vi "Stop Core.vi"(10 "final error code":i32, 11 "Nested in":refnum<class "Valve.lvclass">) -> (3 "Nested out":refnum<class "Valve.lvclass">)   [LabVIEW 2021, in "Valve.lvlib" / "Valve.lvclass"]
doc: "(<B>Filename</B>: Actor Framework.lvlib:Actor.lvclass:Stop Core.vi)\n\nDefines what the actor does before it stops. Use the <B>final error code</B> input to determine whether the actor shut down in response to an error.\n\nBy default, this method does nothing. A descendant class may override it to define behavior, such as shutting down any processes the actor initiated in its override of the Actor Core method."
uses:
  Valve.lvclass
  Valve.lvclass/Valve.ctl
  <vilib>/MGI/Panel Manager/Panel Actor/Panel Actor/Panel Actor.lvclass
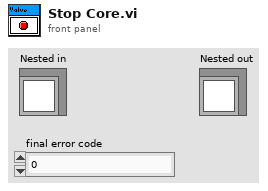
[diagram p1: front panel]
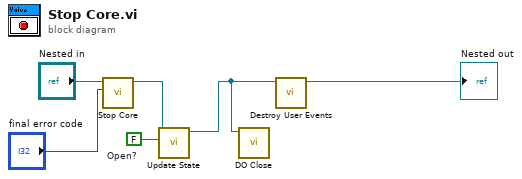
[diagram p0: block diagram]
diagram:
  w1 = FALSE  # Open?
  n1 = call-parent "Stop Core.vi"("final error code"="final error code", "Actor in"="Nested in") -> ("Actor out"=w3:refnum<class "Valve.lvclass">)  [unwired: 9 in]
  n2 = call "Update State.vi"("Open?"=w1, "Valve in"=w3) -> ("Valve out"=w2:refnum<class "Valve.lvclass">)  [unwired: 8 in, 1 out]
  n3 = call "DO Close.vi"("Valve in"=w2) -> ()  [unwired: 10 in, 1 out]
  n4 = call "Destroy User Events.vi"("UI Template in"=w2) -> ("UI Template out"=→"Nested out":refnum<class "Valve.lvclass">)  [unwired: 10 in]
